vi "acquisitionStepByStep.vi"() -> ()   [LabVIEW 2017]
uses:
  globalUtilities.vi
  globalDevices.vi
  <vilib>/Utility/file.llb/Write Delimited Spreadsheet (DBL).vi
panel:
  in  "etlMax(dpt)":dbl
  in  "etlMin(dpt)":dbl
  out "Intensity Graph":u16[][](graph)
  in  "target":bool
  in  "move":i32(ring)=1 items=["1"=1, "2"=2, "etl1"=3]
  out "plane":i32
  in  "bothways":bool
  in  "save volume":bool=TRUE
  out "FINISHED":bool
  in  "# of steps":u16=40
  in  "STOP":bool
  in  "volume height (um)":dbl=20.0
  in  "frames per second":dbl=10.0
  out "folder name":string
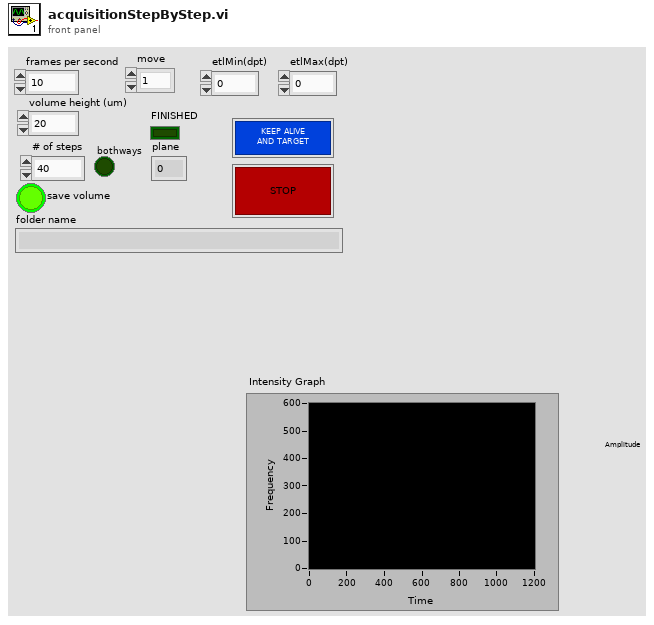
[diagram p1: front panel]
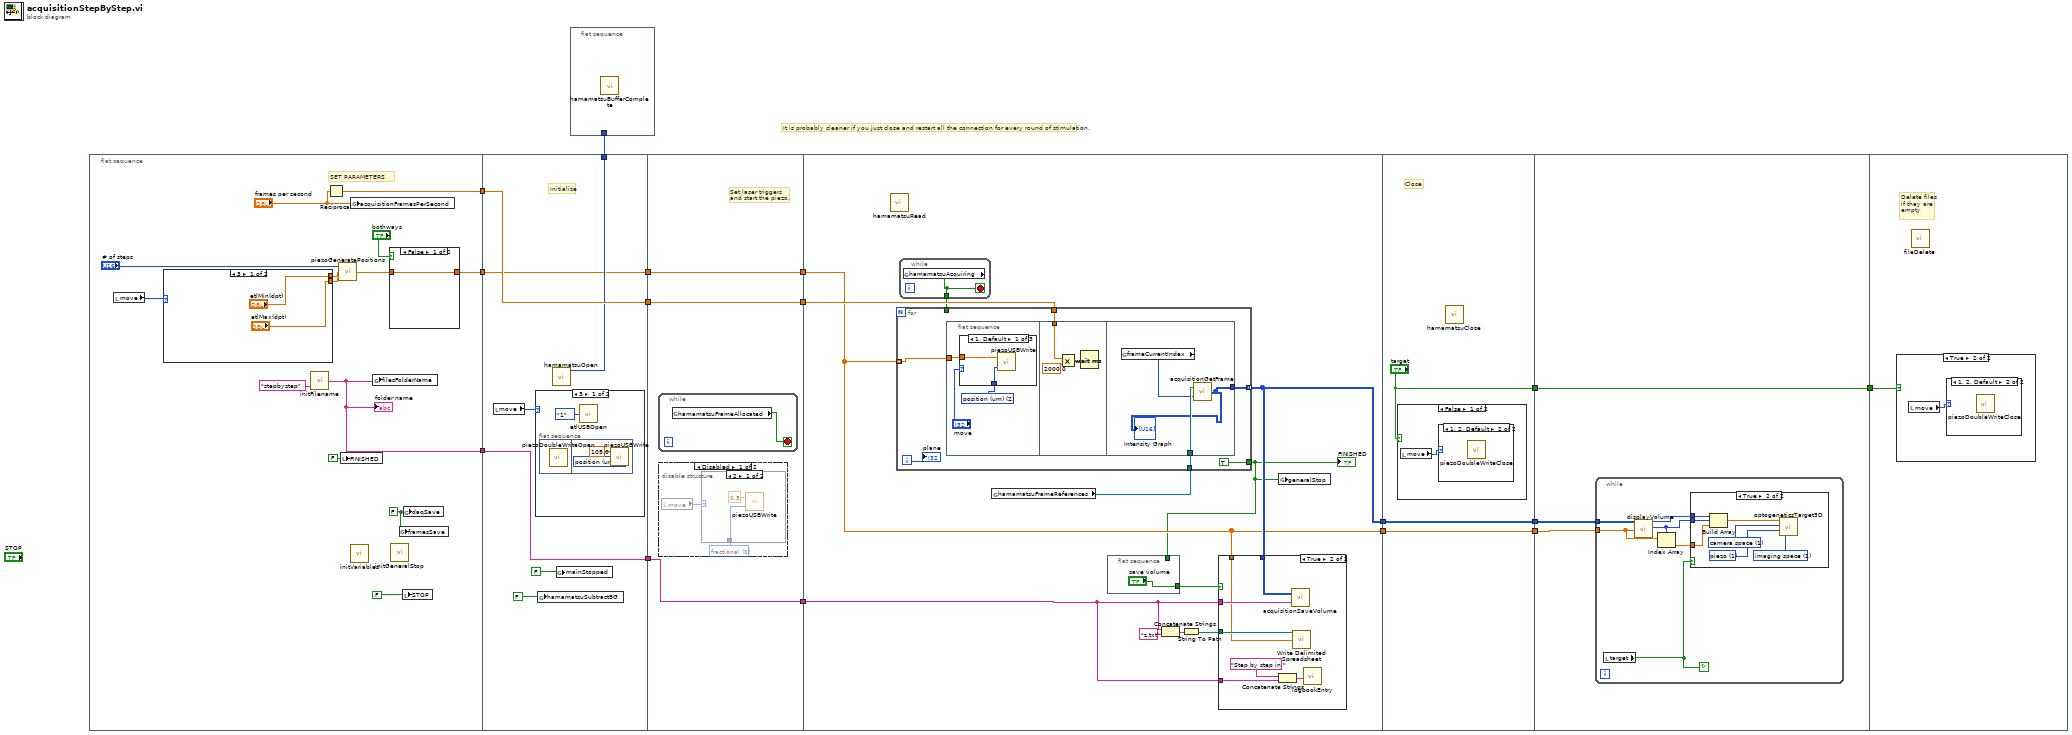
[diagram p0: block diagram]
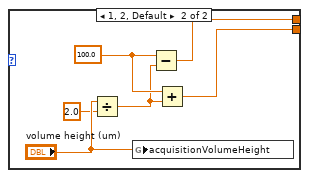
[diagram p2: hidden frame]
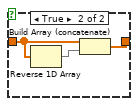
[diagram p3: hidden frame]
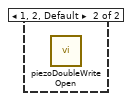
[diagram p4: hidden frame]
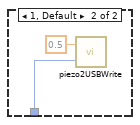
[diagram p5: hidden frame]
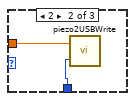
[diagram p8: hidden frame]
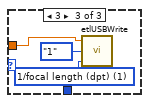
[diagram p9: hidden frame]
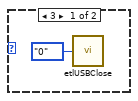
[diagram p10: hidden frame]
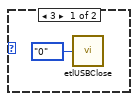
[diagram p14: hidden frame]
diagram:
  # "It is probably cleaner if you just close and restart all the connection for every round of stimulation."
  n1 = flat-sequence {
    tunnel: [w27] -> w16
    tunnel: [w25] -> w9
    tunnel: [w20] -> w7
    tunnel: w16 -> [w47]
    tunnel: [w47] -> w14
    tunnel: [w46] -> w10
    tunnel: w9 -> [w46]
    tunnel: [w45] -> w8
    tunnel: w7 -> [w44]
    tunnel: [w44] -> w5
    tunnel: [w55] -> w15
    tunnel: w14 -> [w55]
    tunnel: [w54] -> w11
    tunnel: w10 -> [w54]
    tunnel: [w53] -> w6
    tunnel: w5 -> [w53]
    tunnel: w15 -> [w73]
    tunnel: [w72] -> w12
    tunnel: w11 -> [w63]
    tunnel: w6 -> [w65]
    tunnel: [w65] -> w3
    tunnel: [w107] -> w13
    tunnel: w12 -> [w107]
    tunnel: [w106] -> w4
    tunnel: w3 -> [w106]
    tunnel: ["target"] -> w2
    tunnel: w13 -> [w112]
    tunnel: w4 -> [w111]
    tunnel: w2 -> [w110]
    tunnel: [w110] -> w1
    tunnel: w1 -> [w126]
    frame #0 {
      w29 = FALSE ("daqSave")
      # "SET PARAMETERS"
      n2 = local read "move"() -> (w17:i32)
      n3 = case shown="3" w17 {
        tunnel: ["etlMin(dpt)" w34] -> w23
        tunnel: ["etlMax(dpt)" w33] -> w22
        frame 3 {
        }
        frame 1, 2, Default {
          w36 = 100.0
          n4 = Divide(x="volume height (um)", y=2.0) -> (x/y=w35:dbl)
          n5 = global write "globalUtilities.vi" "acquisitionVolumeHeight"("volume height (um)") -> ()
          n6 = Subtract(x=w36, y=w35) -> (x-y=w34:dbl)
          n7 = Add(x=w36, y=w35) -> (x+y=w33:dbl)
        }
      }
      n8 = call "initFilename.vi"("Experiment type"="stepbystep") -> ("folder name"=w25:string)  [unwired: 1 in]
      "folder name" <- w25
      n9 = Reciprocal(x="frames per second") -> (1/x=w27:dbl)
      n10 = call "piezoGeneratePositions.vi"("zf"=w22, "z0"=w23, "M"="# of steps") -> ("positions (z)"=w21:dbl[])
      n11 = local write "FINISHED"(FALSE ("Boolean")) -> ()
      n12 = call "initVariables.vi"() -> ()  [unwired: 12 in]
      n13 = global write "globalUtilities.vi" "acquisitionFramesPerSecond"("frames per second") -> ()
      n14 = global write "globalUtilities.vi" "filesFolderName"(w25) -> ()
      n15 = case shown="False" "bothways" {
        tunnel: w21 -> [w39 w41]
        tunnel: [w39 w42] -> w20
        frame False {
        }
        frame True {
          n16 = Reverse 1D Array(array=w41) -> (reversed array=w40:dbl[])
          n17 = Build Array (concatenate)(w41, w40) -> (w42:dbl[])
        }
      }
      n18 = call "initGeneralStop.vi"() -> ()  [unwired: 1 in]
      n19 = global write "globalUtilities.vi" "framesSave"(w29) -> ()
      n20 = local write "STOP"(FALSE) -> ()
      n21 = global write "globalUtilities.vi" "daqSave"(w29) -> ()
    }
    frame #1 {
      # "Initialize"
      n22 = local read "move"() -> (w43:i32)
      n23 = case shown="3" w43 {
        frame 3 {
          n24 = flat-sequence {
            frame #0 {
              n25 = call "piezoDoubleWriteOpen.vi"() -> ()  [unwired: 2 in]
            }
            frame #1 {
              w52 = u16 2 items=["fractional", "voltage (V)", "position (um)"] ("mode")
              n26 = call "piezoUSBWrite.vi"("mode"=w52, "position"=105.0) -> ()  [unwired: 1 in]
            }
          }
          n27 = call "etlUSBOpen.vi"("lens"=enum16{"0", "1"}."1") -> ()  [unwired: 1 in, 1 out]
        }
        frame 1, 2, Default {
          n28 = call "piezoDoubleWriteOpen.vi"() -> ()  [unwired: 2 in]
        }
      }
      n29 = global write "globalDevices.vi" "hamamatsuSubtractBG"(FALSE ("hamamatsuSubtractBG")) -> ()
      n30 = call "hamamatsuOpen.vi"() -> ("Handle out"=w45:u32)  [unwired: 3 out]
      n31 = global write "globalUtilities.vi" "mainStopped"(FALSE ("mainStopped")) -> ()
    }
    frame #2 {
      # "Set laser triggers\nand start the piezo."
      n32 = while {
        stop <- w62 stop-if-true
        n33 = global read "globalDevices.vi" "hamamatsuFrameAllocated"() -> (w62:bool)
      }
      n34 = disable-structure shown="Disabled" {
        frame Disabled {
          w56 = u16 0 items=["fractional", "voltage (V)", "position (um)"] ("mode")
          n35 = local read "move"() -> (w57:i32)
          n36 = case shown="2" w57 {
            tunnel: w56 -> [w58 w60]
            frame 2 {
              n37 = call "piezoUSBWrite.vi"("mode"=w58, "position"=0.5) -> ()  [unwired: 1 in]
            }
            frame 1, Default {
              n38 = call "piezo2USBWrite.vi"("mode"=w60, "position"=0.5) -> ()  [unwired: 1 in]
            }
          }
        }
        frame Enabled {
        }
      }
    }
    frame #3 {
      n39 = call "hamamatsuRead.vi"() -> ()  [unwired: 12 in]
      n40 = while {
        tunnel: [w82] -> w71
        stop <- w82 stop-if-true
        n41 = global read "globalUtilities.vi" "hamamatsuAcquiring"() -> (w82:bool)
      }
      n42 = global read "globalDevices.vi" "hamamatsuFrameReferences"() -> (w70:refnum<data-value>[])
      n43 = for {
        tunnel: w73 -> [w88]
        tunnel: [w87] -> w72 mode=indexing
        tunnel: [TRUE] -> w64
        tunnel: w71 -> [_]
        tunnel: w70 -> [w85]
        tunnel: w65 -> [w84] mode=indexing
        i -> [w83]
        n44 = flat-sequence {
          tunnel: w84 -> [w91]
          tunnel: w88 -> [w101]
          tunnel: [w102] -> w87
          tunnel: w85 -> [w104]
          frame #0 {
            w89 = u16 2 items=["fractional", "voltage (V)", "position (um)"] ("mode")
            n45 = case shown="1, Default" "move" {
              tunnel: w91 -> [w93 w95 w96]
              tunnel: w89 -> [w92 w94 _]
              frame 1, Default {
                n46 = call "piezoUSBWrite.vi"("mode"=w92, "position"=w93) -> ()  [unwired: 1 in]
              }
              frame 2 {
                n47 = call "piezo2USBWrite.vi"("mode"=w94, "position"=w95) -> ()  [unwired: 1 in]
              }
              frame 3 {
                w97 = u16 1 items=["position (um)", "1/focal length (dpt)"] ("mode")
                n48 = call "etlUSBWrite.vi"("mode"=w97, "lens"=enum16{"0", "1"}."1", "input"=w96) -> ()  [unwired: 1 in]
              }
            }
          }
          frame #1 {
            n49 = Multiply(x=w101, y=2000.0) -> (x*y=w99:dbl)
            n50 = Wait (ms)(milliseconds to wait=w99) -> ()  [unwired: 1 out]
          }
          frame #2 {
            n51 = global read "globalUtilities.vi" "frameCurrentIndex"() -> (w103:i32)
            n52 = call "acquisitionGetFrame.vi"("index"=w103, "hamamatsuFrameReferences"=w104) -> ("frameOut"=w102:u16[][])
            "Intensity Graph" <- w102
          }
        }
        "plane" <- w83
      }
      "FINISHED" <- w64
      n53 = flat-sequence {
        tunnel: ["save volume"] -> w69
        tunnel: w64 -> [_]
        frame #0 {
        }
      }
      n54 = Concatenate Strings(w63, "z.txt" ("string")) -> (w67:string)
      n55 = String To Path(string=w67) -> (path=w66:path)
      n56 = case shown="True" w69 {
        tunnel: w72 -> [_ w81]
        tunnel: w63 -> [_ w80]
        tunnel: w66 -> [_ w79]
        tunnel: w65 -> [_ w78]
        tunnel: w63 -> [_ w76]
        frame False {
        }
        frame True {
          n57 = Concatenate Strings("Step by step in " ("Log book entry"), w76) -> (w75:string)
          n58 = call "acquisitionSaveVolume.vi"("folder"=w80, "volume"=w81) -> ()  [unwired: 1 in]
          n59 = call-poly <vilib>:"Write Delimited Spreadsheet.vi"("file path (dialog if empty)"=w79, "1D data"=w78) -> ()  [unwired: 12 in, 2 out]
          n60 = call "logbookEntry.vi"("Log book entry"=w75) -> ()  [unwired: 2 out]
        }
      }
      n61 = global write "globalUtilities.vi" "generalStop"(w64) -> ()
    }
    frame #4 {
      # "Close"
      n62 = case shown="False" "target" {
        frame False {
          n63 = local read "move"() -> (w108:i32)
          n64 = case shown="1, 2, Default" w108 {
            frame 3 {
              n65 = call "etlUSBClose.vi"("lens"=enum16{"0", "1"}."0") -> ()  [unwired: 1 in]
            }
            frame 1, 2, Default {
              n66 = call "piezoDoubleWriteClose.vi"() -> ()  [unwired: 1 in]
            }
          }
        }
        frame True {
        }
      }
      n67 = call "hamamatsuClose.vi"() -> ()  [unwired: 1 out]
    }
    frame #5 {
      n68 = while {
        tunnel: w112 -> [w118]
        tunnel: w111 -> [w115]
        stop <- w117 continue-if-true
        n69 = local read "target"() -> (w117:bool)
        n70 = call "displayVolume.vi"("frames"=w118, "z"=w115) -> ("X0out"=w116:i32, "Y0out"=w114:i32)  [unwired: 12 in, 4 out]
        n71 = Index Array(array=w115, index=w114) -> (element=w113:dbl)
        n72 = case shown="True" w117 {
          tunnel: w116 -> [_ w125]
          tunnel: w114 -> [_ w124]
          tunnel: w113 -> [_ w123]
          frame False {
          }
          frame True {
            w119 = u16 1 items=["optogenetics space", "imaging space"] ("z mode")
            w120 = u16 1 items=["etl", "piezo"] ("z device")
            w121 = u16 1 items=["galvo space", "camera space"] ("xy mode")
            n73 = Build Array(w125, w124, w123) -> (w122:dbl[])
            n74 = call "optogeneticsTarget3D.vi"("z mode"=w119, "z device"=w120, "xy mode"=w121, "xyz"=w122) -> ()  [unwired: 1 in]
          }
        }
      }
    }
    frame #6 {
      # "Delete files\nif they are\nempty"
      n75 = case shown="True" w126 {
        frame False {
        }
        frame True {
          n76 = local read "move"() -> (w127:i32)
          n77 = case shown="1, 2, Default" w127 {
            frame 3 {
              n78 = call "etlUSBClose.vi"("lens"=enum16{"0", "1"}."0") -> ()  [unwired: 1 in]
            }
            frame 1, 2, Default {
              n79 = call "piezoDoubleWriteClose.vi"() -> ()  [unwired: 1 in]
            }
          }
        }
      }
      n80 = call "fileDelete.vi"() -> ()  [unwired: 12 in]
    }
  }
  n81 = flat-sequence {
    tunnel: w8 -> [_]
    frame #0 {
      n82 = call "hamamatsuBufferComplete.vi"() -> ()  [unwired: 12 in]
    }
  }
